vi "motor safety.vi"(0 "Desired Rate":dbl, 1 "Encoder Refnum":string="turret", 5 "Forward Limit":dbl, 9 "Reverse Limit":dbl, 11 "Cutoff Rate":dbl=0.2, 12 "Max Rate":dbl=50.0, 13 "Min Rate":dbl) -> (8 "Rate Output":dbl)   [LabVIEW 2013]
doc: "This VI provides two types of safety for your motors. An encoder for the motor is required. If the encoder reference is innalid, the motor won't be allowed to run. \nThe first safetyis a distance limit. The forward and reverse limit parameters specify the max and min valus for the encoder distance to read until the motor is stopped and only allowed to move away from its limit. \nThe second safety is an encoder safety. The Cutoff Rate parameter is the maximum value allowed to be sent to the motor without a response seen from the encoder. So, if the code is trying to set a value higher than this parameter and the encoder doesn't register a response, the motor will be disabled. It will be reenabled when movement is registered from the encoder. This safety will also permanately disable the motor if the encoder reads some inanely high rate. Consider a replacement...."
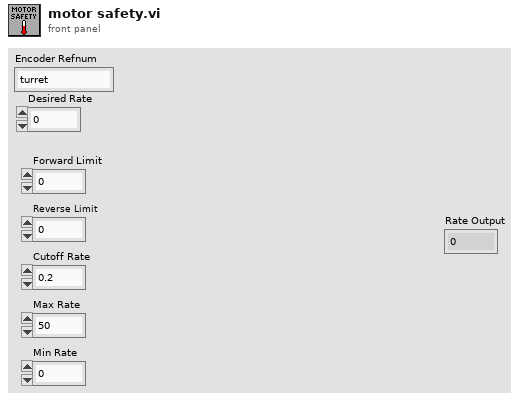
[diagram p1: front panel]
types:
  T1 = typedef "WPI_EncoderDevRef.ctl" = cluster{"DevStatus":errorcluster, "EncoderIndex":T2, "CounterIndex":T3, "DistancePerCount":dbl, "Decoding Type":T4}
  T2 = typedef "FPGA_EncoderIdx.ctl" = enum8{"Enc 0", "Enc 1", "Enc 2", "Enc 3", "Invalid"}
  T3 = typedef "FPGA_CounterCtrSystemIndex.ctl" = enum8{"Ctr 0", "Ctr 1", "Ctr 2", "Ctr 3", "Ctr 4", "Ctr 5", "Ctr 6", "Ctr 7", "Invalid"}
  T4 = typedef "WPI_EncoderType.ctl" = enum16{"1x", "2x", "4x"}
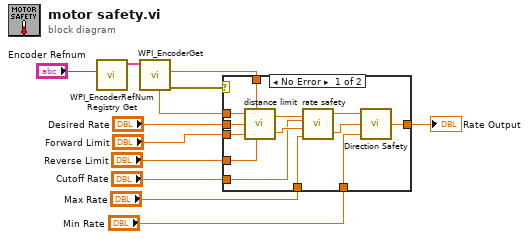
[diagram p0: block diagram]
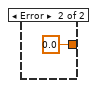
[diagram p2: hidden frame]
diagram:
  n1 = call <vilib>:"WPI_EncoderRefNum Registry Get.vi"("refnum name"="Encoder Refnum") -> ("EncoderDevRef"=w11:T1)  [unwired: 9 in, 1 out]
  n2 = call <vilib>:"WPI_EncoderGet.vi"("EncoderDevRef"=w11) -> ("error out"=w3:errorcluster, "Distance"=w8:dbl, "Rate"=w10:dbl)  [unwired: 5 in, 3 out]
  n3 = case shown="No Error" w3 {
    tunnel: w10 -> [w25 _]
    tunnel: "Desired Rate" -> [w24 _]
    tunnel: w8 -> [w21 _]
    tunnel: [w13 0.0 ("Output Rate")] -> w7
    tunnel: "Forward Limit" -> [w20 _]
    tunnel: "Reverse Limit" -> [w19 _]
    tunnel: "Cutoff Rate" -> [w18 _]
    tunnel: "Max Rate" -> [w17 _]
    tunnel: "Min Rate" -> [w14 _]
    frame No Error {
      n4 = call "distance limit.vi"("Encoder Rate"=w25, "Encoder Distance"=w21, "Desired Rate"=w24, "Forward Limit"=w20, "Reverse Limit"=w19) -> ("Encoder Rate Out"=w23:dbl, "Output Rate"=w22:dbl)
      n5 = call "rate safety.vi"("Max Rate"=w17, "Desired Rate"=w22, "Cutoff Rate"=w18, "Encoder Rate"=w23) -> ("Output Rate"=w15:dbl, "Encoder Rate Out"=w16:dbl)
      n6 = call "Direction Safety.vi"("Min Rate"=w14, "Desired Rate"=w15, "Encoder Rate"=w16) -> ("Super Safe Rate"=w13:dbl)
    }
    frame Error {
    }
  }
  "Rate Output" <- w7
